vi "Read OPC ini param.vi"(8 "error in (no error)":errorcluster, 9 "configuration file path":path, 10 "key":string="Server", 11 "Server in":T1) -> (0 "error out":errorcluster, 3 "Server out":T1)   [LabVIEW 2019, in "OPC addons.lvlib"]
uses:
  OPC addons.lvlib
  <vilib>/Utility/config.llb/Read Key (String).vi
  <vilib>/Utility/config.llb/NI_LVConfig.lvlib
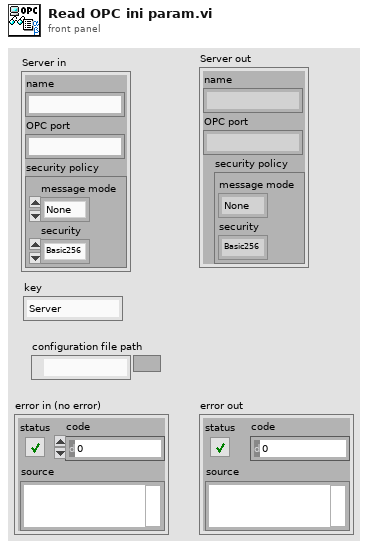
[diagram p1: front panel]
types:
  T1 = cluster{"name":string, "OPC port":string, "security policy":cluster{"message mode":enum16{"None", "Sign", "Sign and Encrypt"}, "security":enum16{"Basic256", "Basic128Rsa15"}}}
  T2 = typedef "NI_LVConfig.lvlib/Config Data RefNum.ctl" = refnum<k1>
  T3 = cluster{"[0]":string, "[1]":string, "[2]":string, "[3]":string}
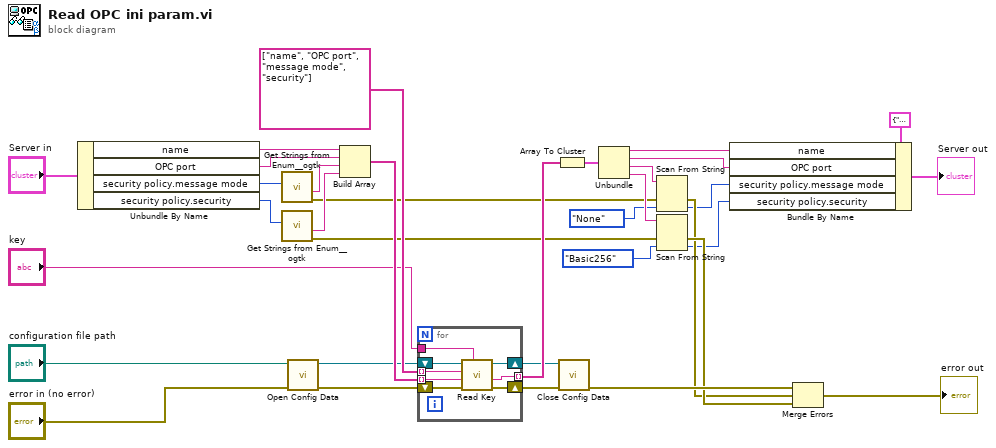
[diagram p0: block diagram]
diagram:
  n1 = Unbundle By Name("Server in") -> ("name"=w25:string, "OPC port"=w26:string, "security policy.message mode"=w3:enum16{"None", "Sign", "Sign and Encrypt"}, "security policy.security"=w4:enum16{"Basic256", "Basic128Rsa15"})
  n2 = call <userlib>:"Get Strings from Enum__ogtk.vi"("Enum"=w3) -> ("error out"=w8:errorcluster, "String Value"=w27:string)  [unwired: 7 in, 2 out]
  n3 = call <userlib>:"Get Strings from Enum__ogtk.vi"("Enum"=w4) -> ("error out"=w7:errorcluster, "String Value"=w28:string)  [unwired: 7 in, 2 out]
  n4 = call <vilib>:"Open Config Data.vi"("error in (no error)"="error in (no error)", "configuration file path"="configuration file path") -> ("error out"=w21:errorcluster, "refnum"=w20:T2)  [unwired: 7 in, 1 out]
  n5 = Build Array(w25, w26, w27, w28) -> (w29:string[])
  n6 = for {
    tunnel: "key" -> [w39]
    tunnel: w29 -> [w37] mode=indexing
    shift-right: [w36] -> w17
    shift-left: w21 -> [w42]
    shift-right: [w35] -> w16
    shift-left: w20 -> [w41]
    tunnel: string[] ["name", "OPC port", "message mode", "security"] -> [w40] mode=indexing
    tunnel: [w38] -> w19 mode=indexing
    n7 = call-poly <vilib>:"Read Key.vi"("section"=w39, "error in (no error)"=w42, "default value"=w37, "key"=w40, "refnum"=w41) -> ("error out"=w36:errorcluster, "value"=w38:string, "refnum out"=w35:T2)  [unwired: 3 in, 1 out]
  }
  n8 = Array To Cluster(array=w19) -> (cluster=w18:T3)
  n9 = call <vilib>:"Close Config Data.vi"("error in (no error)"=w17, "refnum"=w16) -> ("error out"=w34:errorcluster)  [unwired: 8 in, 1 out]
  n10 = Unbundle(w18) -> ("[0]"=w32:string, "[1]"=w33:string, "[2]"=w30:string, "[3]"=w31:string)
  n11 = Scan From String(input string=w30, error in=w8, default 1=enum16{"None", "Sign", "Sign and Encrypt"}."None" ("Server.security policy.message mode")) -> (error out=w14:errorcluster, output 1=w13:enum16{"None", "Sign", "Sign and Encrypt"})  [unwired: 2 in, 2 out]
  n12 = Scan From String(input string=w31, error in=w7, default 1=enum16{"Basic256", "Basic128Rsa15"}."Basic256" ("Server.security policy.security")) -> (error out=w15:errorcluster, output 1=w12:enum16{"Basic256", "Basic128Rsa15"})  [unwired: 2 in, 2 out]
  n13 = Bundle By Name(cluster=T1 {"name"="H1", "OPC port"="49580", "security policy"={"message mode"=enum."None", "security"=enum."Basic256"}} ("Server"), "name"=w32, "OPC port"=w33, "security policy.message mode"=w13, "security policy.security"=w12) -> (→"Server out":T1)
  n14 = Merge Errors(w34, w14, w15) -> (→"error out":errorcluster)
